vi "Download Files From HTTPS.vi"(0 "current version":string, 2 "download firmware?":bool=TRUE, 7 "GUI search key":string="###FIRMWARE_DOWNLOAD_ALL###") -> (8 "updated":bool)   [LabVIEW 2010]
uses:
  <vilib>/Utility/sysdir.llb/System Directory Type.ctl
  <vilib>/zip/NI_Unzip.lvlib
panel:
  out "Not Used 2":bool caption="(it may take some minutes)"
  out "Not Used":bool caption="Checking for updates"
  out "major current":i32
  out "minor current":i32
  out "patch current":i32
  out "patch":i32
  out "minor":i32
  out "major":i32
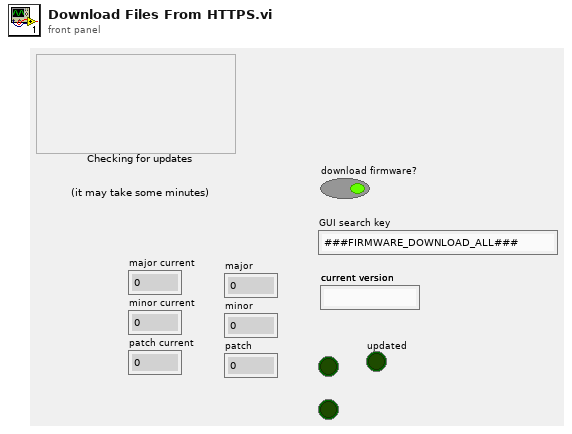
[diagram p1: front panel]
types:
  T1 = typedef "System Directory Type.ctl" = i32
  T2 = enum16{"open", "replace", "create", "open or create", "replace or create", "replace or create with confirmation"}
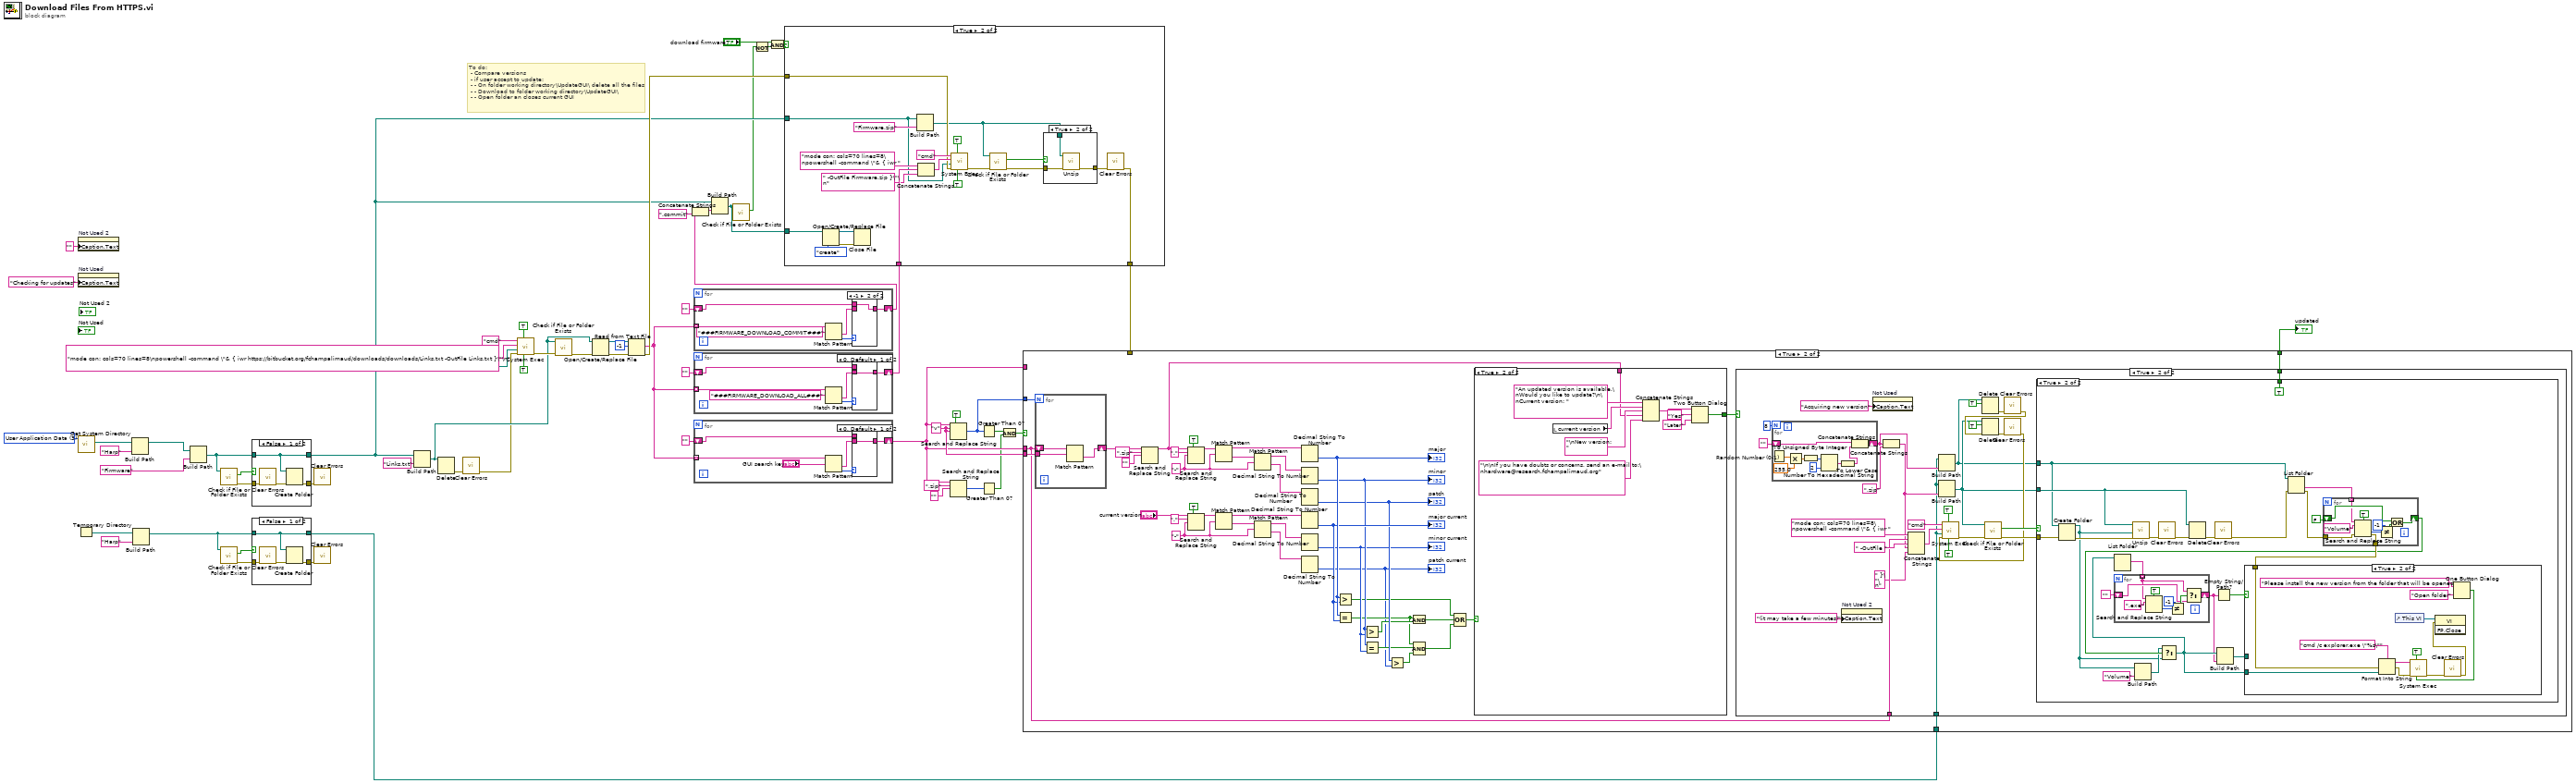
[diagram p0: block diagram]
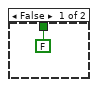
[diagram p6: hidden frame]
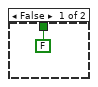
[diagram p7: hidden frame]
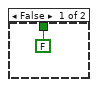
[diagram p8: hidden frame]
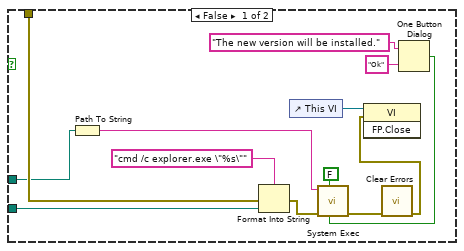
[diagram p9: hidden frame]
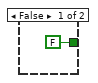
[diagram p10: hidden frame]
diagram:
  w21 = T1 3 items=["User Home"=0, "User Desktop"=1, "User Documents"=2, "User Application Data"=3, "User Preferences"=4, "User Temporary"=5, "Public Documents"=6, "Public Application Data"=7, "Public Preferences"=8, "Public Cache"=13, "System Core Libraries"=9, "System Installed Libraries"=10, "Application Files"=11, "Boot Volume Root"=12] ("system directory type")
  w38 = "v" ("search string")
  # "To do:\n - Compare versions\n - if user accept to update:\n - - On folder working directory\\UpdateGUI\\ delete all the files\n - - Download to folder working directory\\UpdateGUI\\\n - - Open folder an closes current GUI"
  n1 = call <vilib>:"Get System Directory.vi"("system directory type"=w21) -> ("system directory"=w20:path)  [unwired: 10 in]
  n2 = Temporary Directory() -> (w16:path)
  n3 = property on="Not Used 2" class="Bool (strict)"("Caption.Text"="") -> ()  [unwired: 2 in, 2 out]
  n4 = property on="Not Used" class="Bool (strict)"("Caption.Text"="Checking for updates") -> ()  [unwired: 2 in, 2 out]
  n5 = Build Path(base path=w20, name or relative path="Harp") -> (appended path=w19:path)
  n6 = Build Path(base path=w16, name or relative path="Harp") -> (appended path=w15:path)
  n7 = Build Path(base path=w19, name or relative path="Firmware") -> (appended path=w17:path)
  n8 = call <vilib>:"Check if File or Folder Exists.vi"("path"=w17) -> ("error out"=w43:errorcluster, "file or folder exists?"=w41:bool)  [unwired: 8 in, 1 out]
  n9 = call <vilib>:"Check if File or Folder Exists.vi"("path"=w15) -> ("error out"=w28:errorcluster, "file or folder exists?"=w30:bool)  [unwired: 8 in, 1 out]
  n10 = case shown="False" w41 {
    tunnel: w17 -> [w59 w63]
    tunnel: w43 -> [w62 w64]
    tunnel: [w60 w64] -> w42
    tunnel: [w59 w63] -> w9
    frame False {
      n11 = call <vilib>:"Clear Errors.vi"("error in (no error)"=w62) -> ("error out"=w61:errorcluster)  [unwired: 6 in]
      n12 = Create Folder(path (use dialog)=w59, error in=w61) -> (error out=w60:errorcluster)  [unwired: 1 in, 2 out]
    }
    frame True {
    }
  }
  n13 = case shown="False" w30 {
    tunnel: w15 -> [w65 w69]
    tunnel: w28 -> [w68 w70]
    tunnel: [w66 w70] -> w29
    tunnel: [w65 w69] -> w27
    frame False {
      n14 = call <vilib>:"Clear Errors.vi"("error in (no error)"=w68) -> ("error out"=w67:errorcluster)  [unwired: 6 in]
      n15 = Create Folder(path (use dialog)=w65, error in=w67) -> (error out=w66:errorcluster)  [unwired: 1 in, 2 out]
    }
    frame True {
    }
  }
  n16 = call <vilib>:"Clear Errors.vi"("error in (no error)"=w42) -> ()  [unwired: 6 in, 1 out]
  n17 = call <vilib>:"Clear Errors.vi"("error in (no error)"=w29) -> ()  [unwired: 6 in, 1 out]
  n18 = Build Path(base path=w9, name or relative path="Links.txt") -> (appended path=w51:path)
  n19 = Delete(path (use dialog)=w51) -> (error out=w54:errorcluster)  [unwired: 4 in, 2 out]
  n20 = call <vilib>:"Clear Errors.vi"("error in (no error)"=w54) -> ("error out"=w4:errorcluster)  [unwired: 6 in]
  n21 = call <vilib>:"System Exec.vi"("run minimized? (F)"=TRUE, "wait until completion? (T)"=TRUE, "error in (no error)"=w4, "working directory"=w9, "standard input"="mode con: cols=70 lines=8\npowershell -command \"& { iwr https://bitbucket.org/fchampalimaud/downloads/downloads/Links.txt -OutFile Links.txt }\"\n", "command line"="cmd") -> ("error out"=w53:errorcluster)  [unwired: 2 in, 3 out]
  n22 = call <vilib>:"Check if File or Folder Exists.vi"("error in (no error)"=w53, "path"=w51) -> ("error out"=w3:errorcluster)  [unwired: 7 in, 2 out]
  n23 = Open/Create/Replace File(file path (use dialog)=w51, error in=w3) -> (refnum out=w48:refnum<file>, error out=w50:errorcluster)  [unwired: 4 in, 1 out]
  n24 = Read from Text File(file (use dialog)=w48, count=-1, error in=w50) -> (text=w13:string[], error out=w44:errorcluster)  [unwired: 1 in, 2 out]
  n25 = for {
    tunnel: w13 -> [w76] mode=indexing
    shift-right: [w72] -> w11
    shift-left: "" -> [w71]
    n26 = Match Pattern(string=w76, regular expression="###FIRMWARE_DOWNLOAD_COMMIT###" ("search string")) -> (after substring=w73:string, offset past match=w74:i32)  [unwired: 1 in, 2 out]
    n27 = case shown="-1" w74 {
      tunnel: w73 -> [w77 _]
      tunnel: [w77 w78] -> w72
      tunnel: w71 -> [_ w78]
      frame 0, Default {
      }
      frame -1 {
      }
    }
  }
  n28 = Concatenate Strings(w11, ".commit" ("string")) -> (w10:string)
  n29 = for {
    tunnel: w13 -> [w84] mode=indexing
    shift-right: [w80] -> w45
    shift-left: "" -> [w79]
    n30 = Match Pattern(string=w84, regular expression="###FIRMWARE_DOWNLOAD_ALL###" ("search string")) -> (after substring=w81:string, offset past match=w82:i32)  [unwired: 1 in, 2 out]
    n31 = case shown="0, Default" w82 {
      tunnel: w81 -> [w85 _]
      tunnel: [w85 w86] -> w80
      tunnel: w79 -> [_ w86]
      frame 0, Default {
      }
      frame -1 {
      }
    }
  }
  n32 = for {
    tunnel: w13 -> [w92] mode=indexing
    shift-right: [w88] -> w34
    shift-left: "" -> [w87]
    n33 = Match Pattern(string=w92, regular expression="GUI search key") -> (after substring=w89:string, offset past match=w90:i32)  [unwired: 1 in, 2 out]
    n34 = case shown="0, Default" w90 {
      tunnel: w89 -> [w93 _]
      tunnel: [w93 w94] -> w88
      tunnel: w87 -> [_ w94]
      frame 0, Default {
      }
      frame -1 {
      }
    }
  }
  n35 = Build Path(base path=w9, name or relative path=w10) -> (appended path=w5:path)
  n36 = call <vilib>:"Check if File or Folder Exists.vi"("path"=w5) -> ("file or folder exists?"=w7:bool)  [unwired: 8 in, 2 out]
  n37 = Not(x=w7) -> (.not. x?=w6:bool)
  n38 = And(x="download firmware?", y=w6) -> (x .and. y?=w8:bool)
  n39 = case shown="True" w8 {
    tunnel: w45 -> [_ w115]
    tunnel: w44 -> [w95 w106]
    tunnel: w9 -> [_ w101]
    tunnel: [w95 w100] -> w2
    tunnel: w5 -> [_ w99]
    frame False {
    }
    frame True {
      n40 = Open/Create/Replace File(file path (use dialog)=w99, operation (0:open)=T2."create") -> (refnum out=w96:refnum<file>, error out=w97:errorcluster)  [unwired: 4 in, 1 out]
      n41 = Close File(refnum=w96, error in=w97) -> ()  [unwired: 2 out]
      n42 = Build Path(base path=w101, name or relative path="Firmware.zip") -> (appended path=w102:path)
      n43 = Concatenate Strings("mode con: cols=70 lines=8\npowershell -command \"& { iwr " ("standard input"), w115, " -OutFile Firmware.zip }\"\n" ("standard input")) -> (w108:string)
      n44 = call <vilib>:"System Exec.vi"("run minimized? (F)"=TRUE, "wait until completion? (T)"=TRUE, "error in (no error)"=w106, "working directory"=w101, "standard input"=w108, "command line"="cmd") -> ("error out"=w111:errorcluster)  [unwired: 2 in, 3 out]
      n45 = call <vilib>:"Check if File or Folder Exists.vi"("error in (no error)"=w111, "path"=w102) -> ("error out"=w104:errorcluster, "file or folder exists?"=w105:bool)  [unwired: 7 in, 1 out]
      n46 = case shown="True" w105 {
        tunnel: w102 -> [_ w119]
        tunnel: w104 -> [w116 w118]
        tunnel: [w116 w117] -> w103
        frame False {
        }
        frame True {
          n47 = call <vilib>:"Unzip.vi"("error in (no error)"=w118, "Zip file"=w119) -> ("error out"=w117:errorcluster)  [unwired: 7 in, 2 out]
        }
      }
      n48 = call <vilib>:"Clear Errors.vi"("error in (no error)"=w103) -> ("error out"=w100:errorcluster)  [unwired: 6 in]
    }
  }
  n49 = Search and Replace String(replace all?=TRUE ("replace all? (F)"), input string=w34, search string=w38, replace string=w38) -> (number of replacements=w39:i32)  [unwired: 4 in, 3 out]
  n50 = Search and Replace String(input string=w34, search string=".zip", replace string="" ("replace string (\"\")")) -> (number of replacements=w33:i32)  [unwired: 5 in, 3 out]
  n51 = Greater Than 0?(x=w39) -> (x > 0?=w37:bool)
  n52 = Greater Than 0?(x=w33) -> (x > 0?=w31:bool)
  n53 = And(x=w37, y=w31) -> (x .and. y?=w32:bool)
  n54 = case shown="True" w32 {
    tunnel: w39 -> [_ w161]
    tunnel: w34 -> [_ w126]
    tunnel: w38 -> [_ w160]
    tunnel: w34 -> [_ _]
    tunnel: w27 -> [_ w124]
    tunnel: [FALSE ("true") w123] -> w25
    tunnel: w2 -> [_ _]
    frame False {
    }
    frame True {
      w148 = "-" ("search string")
      w152 = "-" ("search string")
      n55 = for {
        N: w161 -> [_]
        shift-right: [w278] -> w151
        shift-left: w126 -> [w279]
        tunnel: w160 -> [w277]
        n56 = Match Pattern(string=w279, regular expression=w277) -> (after substring=w278:string)  [unwired: 1 in, 3 out]
      }
      n57 = Search and Replace String(input string=w151, search string=".zip", replace string="" ("replace string (\"\")")) -> (result string=w127:string)  [unwired: 5 in, 3 out]
      n58 = Search and Replace String(replace all?=TRUE ("replace all? (F)"), input string=w127, search string=".", replace string=w152) -> (result string=w158:string)  [unwired: 4 in, 3 out]
      n59 = Search and Replace String(replace all?=TRUE ("replace all? (F)"), input string="current version", search string=".", replace string=w148) -> (result string=w142:string)  [unwired: 4 in, 3 out]
      n60 = Match Pattern(string=w158, regular expression=w152) -> (before substring=w155:string, after substring=w157:string)  [unwired: 1 in, 2 out]
      n61 = Match Pattern(string=w142, regular expression=w148) -> (before substring=w145:string, after substring=w143:string)  [unwired: 1 in, 2 out]
      n62 = Match Pattern(string=w157, regular expression=w152) -> (before substring=w154:string, after substring=w153:string)  [unwired: 1 in, 2 out]
      n63 = Match Pattern(string=w143, regular expression=w148) -> (before substring=w146:string, after substring=w147:string)  [unwired: 1 in, 2 out]
      n64 = Decimal String To Number(string=w155) -> (number=w139:i32)  [unwired: 2 in, 1 out]
      "major" <- w139
      n65 = Decimal String To Number(string=w154) -> (number=w137:i32)  [unwired: 2 in, 1 out]
      "minor" <- w137
      n66 = Decimal String To Number(string=w153) -> (number=w136:i32)  [unwired: 2 in, 1 out]
      "patch" <- w136
      n67 = Decimal String To Number(string=w145) -> (number=w138:i32)  [unwired: 2 in, 1 out]
      "major current" <- w138
      n68 = Decimal String To Number(string=w146) -> (number=w135:i32)  [unwired: 2 in, 1 out]
      "minor current" <- w135
      n69 = Decimal String To Number(string=w147) -> (number=w122:i32)  [unwired: 2 in, 1 out]
      "patch current" <- w122
      n70 = Greater?(x=w139, y=w138) -> (0:w130:bool)
      n71 = Equal?(x=w139, y=w138) -> (x = y?=w131:bool)
      n72 = Greater?(x=w137, y=w135) -> (0:w134:bool)
      n73 = Equal?(x=w137, y=w135) -> (x = y?=w133:bool)
      n74 = Greater?(x=w136, y=w122) -> (0:w132:bool)
      n75 = And(x=w131, y=w134) -> (x .and. y?=w129:bool)
      n76 = Compound Arithmetic op=AND(w131, w133, w132) -> (w128:bool)
      n77 = Compound Arithmetic op=OR(w130, w129, w128) -> (w121:bool)
      n78 = case shown="True" w121 {
        tunnel: w127 -> [_ w273]
        tunnel: [FALSE ("T button?") w269] -> w125
        frame False {
        }
        frame True {
          n79 = local read "current version"() -> (w275:string)
          n80 = Concatenate Strings("An updated version is available.\nWould you like to update?\n\nCurrent version: " ("message"), w275, "\nNew version: " ("message"), w273, "\n\nIf you have doubts or concerns, send an e-mail to:\nhardware@research.fchampalimaud.org" ("string")) -> (w272:string)
          n81 = Two Button Dialog(message=w272, 1:"Later" ("F button name (\"Cancel\")"), 2:"Yes" ("T button name (\"OK\")")) -> (T button?=w269:bool)
        }
      }
      n82 = case shown="True" w125 {
        tunnel: w126 -> [_ w184]
        tunnel: w124 -> [_ w164]
        tunnel: [FALSE ("true") w179] -> w123
        frame False {
        }
        frame True {
          n83 = for {
            N: 8 ("Numeric") -> [_]
            shift-right: [w193] -> w166
            shift-left: "" -> [w191]
            n84 = Random Number (0-1)() -> (number: 0 to 1=w199:dbl)
            n85 = Multiply(x=w199, y=255.0) -> (x*y=w197:dbl)
            n86 = To Unsigned Byte Integer(number=w197) -> (unsigned 8bit integer=w196:u8)
            n87 = Number To Hexadecimal String(1:i16 2 ("width (-)"), 2:w196) -> (0:w194:string)
            n88 = To Lower Case(string=w194) -> (all lower case string=w192:string)
            n89 = Concatenate Strings(w191, w192) -> (w193:string)
          }
          n90 = property on="Not Used 2" class="Bool (strict)"("Caption.Text"="(it may take a few minutes)") -> ()  [unwired: 2 in, 2 out]
          n91 = property on="Not Used" class="Bool (strict)"("Caption.Text"="Acquiring new version") -> ()  [unwired: 2 in, 2 out]
          n92 = Concatenate Strings(w166, ".zip" ("string")) -> (w173:string)
          n93 = Concatenate Strings("mode con: cols=70 lines=8\npowershell -command \"& { iwr " ("standard input"), w184, " -OutFile " ("standard input"), w173, " }\"\n" ("standard input")) -> (w190:string)
          n94 = Build Path(base path=w164, name or relative path=w166) -> (appended path=w165:path)
          n95 = Build Path(base path=w164, name or relative path=w173) -> (appended path=w167:path)
          n96 = Delete(path (use dialog)=w165, entire hierarchy (F)=TRUE) -> (error out=w175:errorcluster)  [unwired: 3 in, 2 out]
          n97 = call <vilib>:"Clear Errors.vi"("error in (no error)"=w175) -> ("error out"=w168:errorcluster)  [unwired: 6 in]
          n98 = Delete(path (use dialog)=w167, entire hierarchy (F)=TRUE, error in=w168) -> (error out=w170:errorcluster)  [unwired: 2 in, 2 out]
          n99 = call <vilib>:"Clear Errors.vi"("error in (no error)"=w170) -> ("error out"=w169:errorcluster)  [unwired: 6 in]
          n100 = call <vilib>:"System Exec.vi"("run minimized? (F)"=TRUE, "wait until completion? (T)"=TRUE, "error in (no error)"=w169, "working directory"=w164, "standard input"=w190, "command line"="cmd") -> ("error out"=w183:errorcluster)  [unwired: 2 in, 3 out]
          n101 = call <vilib>:"Check if File or Folder Exists.vi"("error in (no error)"=w183, "path"=w167) -> ("error out"=w182:errorcluster, "file or folder exists?"=w181:bool)  [unwired: 7 in, 1 out]
          n102 = case shown="True" w181 {
            tunnel: w182 -> [_ w223]
            tunnel: w167 -> [_ w222]
            tunnel: [FALSE ("true") TRUE ("true")] -> w179
            tunnel: w165 -> [_ w215]
            frame False {
            }
            frame True {
              n103 = Create Folder(path (use dialog)=w215, error in=w223) -> (created path=w210:path, error out=w218:errorcluster)  [unwired: 1 in, 1 out]
              n104 = call <vilib>:"Unzip.vi"("error in (no error)"=w218, "Target directory (same as Zip file if empty)"=w210, "Zip file"=w222) -> ("error out"=w221:errorcluster)  [unwired: 6 in, 2 out]
              n105 = Build Path(base path=w210, name or relative path="Volume") -> (appended path=w211:path)
              n106 = call <vilib>:"Clear Errors.vi"("error in (no error)"=w221) -> ("error out"=w220:errorcluster)  [unwired: 6 in]
              n107 = Delete(path (use dialog)=w222, error in=w220) -> (error out=w219:errorcluster)  [unwired: 3 in, 2 out]
              n108 = call <vilib>:"Clear Errors.vi"("error in (no error)"=w219) -> ("error out"=w209:errorcluster)  [unwired: 6 in]
              n109 = List Folder(path=w215, error in=w209) -> (folder names=w216:string[], error out=w208:errorcluster)  [unwired: 2 in, 2 out]
              n110 = for {
                shift-right: [w236] -> w212
                shift-left: FALSE -> [w235]
                tunnel: w216 -> [w234] mode=indexing
                tunnel: w208 -> [w233]
                tunnel: [w232] -> w214
                n111 = Search and Replace String(case sensitive?=TRUE ("ignore case? (F)"), input string=w234, search string="Volume", error in=w233) -> (offset past replacement=w238:i32, error out=w232:errorcluster)  [unwired: 4 in, 2 out]
                n112 = Not Equal?(x=-1, y=w238) -> (x != y?=w241:bool)
                n113 = Or(x=w235, y=w241) -> (x .or. y?=w236:bool)
              }
              n114 = Select(t=w211, s=w212, f=w210) -> (s? t:f=w205:path)
              n115 = List Folder(path=w205) -> (filenames=w206:string[])  [unwired: 3 in, 3 out]
              n116 = for {
                shift-right: [w224] -> w204
                shift-left: "" -> [w226]
                tunnel: w206 -> [w225] mode=indexing
                n117 = Search and Replace String(case sensitive?=TRUE ("ignore case? (F)"), input string=w225, search string=".exe") -> (offset past replacement=w229:i32)  [unwired: 5 in, 3 out]
                n118 = Not Equal?(x=-1, y=w229) -> (x != y?=w227:bool)
                n119 = Select(t=w225, s=w227, f=w226) -> (s? t:f=w224:string)
              }
              n120 = Empty String/Path?(string/path=w204) -> (empty?=w203:bool)
              n121 = Build Path(base path=w205, name or relative path=w204) -> (appended path=w201:path)
              n122 = case shown="True" w203 {
                tunnel: w205 -> [w244 w261]
                tunnel: w214 -> [w248 w259]
                tunnel: w201 -> [w246 _]
                frame False {
                  n123 = Path To String(path=w246) -> (string=w245:string)
                  n124 = Format Into String(format string="cmd /c explorer.exe \"%s\"", error in=w248, w244) -> (error out=w253:errorcluster)  [unwired: 1 in, 1 out]
                  n125 = control-ref of="This VI"() -> (w254:refnum<vi>)
                  n126 = One Button Dialog(message="The new version will be installed.", button name ("OK")="Ok") -> (true=w243:bool)
                  n127 = call <vilib>:"System Exec.vi"("run minimized? (F)"=w243, "wait until completion? (T)"=FALSE, "error in (no error)"=w253, "command line"=w245) -> ("error out"=w252:errorcluster)  [unwired: 4 in, 3 out]
                  n128 = call <vilib>:"Clear Errors.vi"("error in (no error)"=w252) -> ("error out"=w250:errorcluster)  [unwired: 6 in]
                  n129 = invoke class="VI" method="FP.Close"(reference=w254, error in=w250) -> ()  [unwired: 1 in, 3 out]
                }
                frame True {
                  n130 = Format Into String(format string="cmd /c explorer.exe \"%s\"", error in=w259, w261) -> (resulting string=w265:string, error out=w264:errorcluster)  [unwired: 1 in]
                  n131 = control-ref of="This VI"() -> (w266:refnum<vi>)
                  n132 = One Button Dialog(message="Please install the new version from the folder that will be opened.", button name ("OK")="Open folder") -> (true=w256:bool)
                  n133 = call <vilib>:"System Exec.vi"("run minimized? (F)"=w256, "wait until completion? (T)"=TRUE, "error in (no error)"=w264, "command line"=w265) -> ("error out"=w263:errorcluster)  [unwired: 4 in, 3 out]
                  n134 = call <vilib>:"Clear Errors.vi"("error in (no error)"=w263) -> ("error out"=w260:errorcluster)  [unwired: 6 in]
                  n135 = invoke class="VI" method="FP.Close"(reference=w266, error in=w260) -> ()  [unwired: 1 in, 3 out]
                }
              }
            }
          }
        }
      }
    }
  }
  "updated" <- w25
